vi "SensorInfo.vi"(0 "Serial Number":string, 5 "Family":u16(ring) items=["Iris Slim", "Iris Compact", "Iris xxxx"], 9 "Revision (iteración)":string) -> (4 "Serial Number out":string, 6 "Family out":u16(ring) items=["Iris Slim", "Iris xxxx", "Iris xxxx"], 8 "Part Number out":string, 10 "Revision out":string)   [LabVIEW 2018]
panel:
  in  "Cancel":bool
  in  "OK":bool
  # "Test Information"
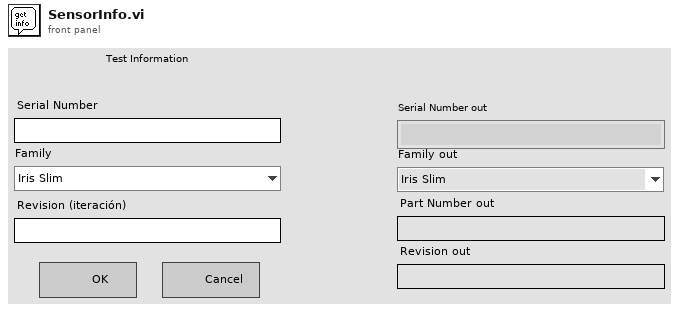
[diagram p1: front panel]
types:
  T1 = enum8{"Enabled", "Disabled", "Disabled and Grayed Out"}
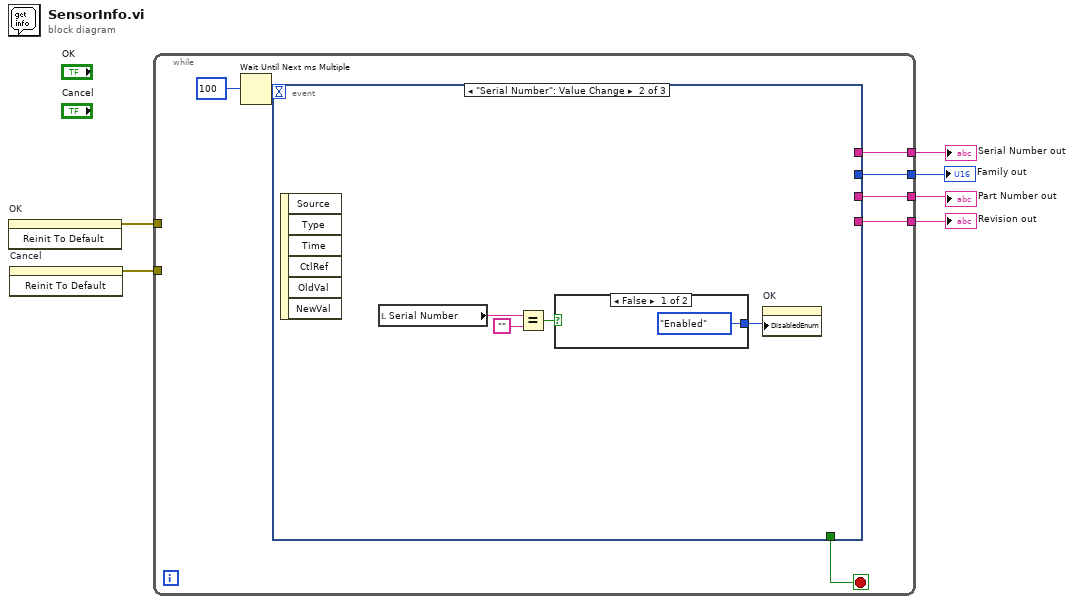
[diagram p0: block diagram]
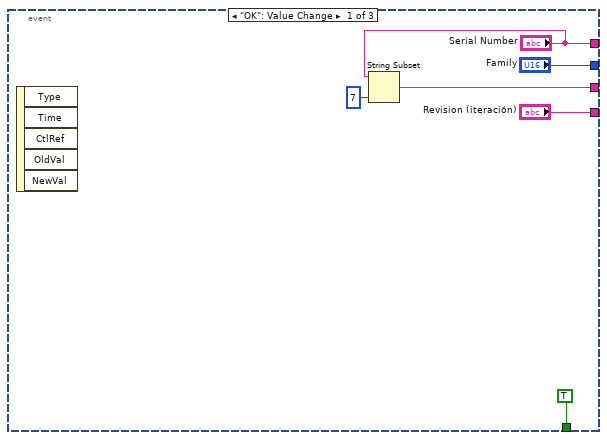
[diagram p2: hidden frame]
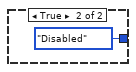
[diagram p3: hidden frame]
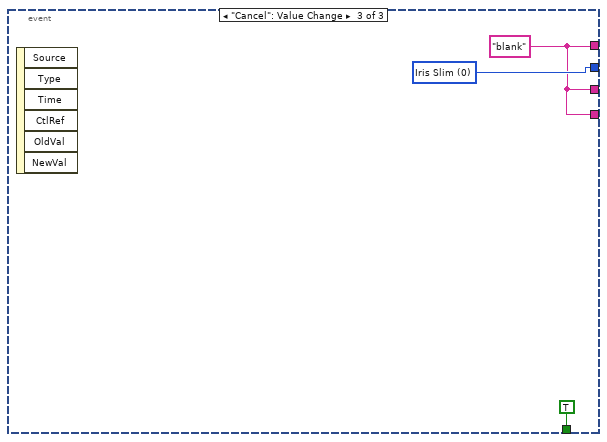
[diagram p4: hidden frame]
diagram:
  n1 = invoke on="OK" class="Bool" method="Reinit To Default"() -> (error out=w5:errorcluster)  [unwired: 3 in, 2 out]
  n2 = invoke on="Cancel" class="Bool" method="Reinit To Default"() -> (error out=w4:errorcluster)  [unwired: 3 in, 2 out]
  n3 = while {
    tunnel: [w12] -> w6
    tunnel: [w11] -> w1
    tunnel: w5 -> [_]
    tunnel: w4 -> [_]
    tunnel: [w8] -> w3
    tunnel: [w7] -> w2
    stop <- w9 stop-if-true
    n4 = Wait Until Next ms Multiple(millisecond multiple=100) -> ()  [unwired: 1 out]
    n5 = event shown="[1] \"Serial Number\": Value Change" {
      selector: _ -> [_ _ _]
      dyn-events: _ -> [_ _ _]
      timeout: _ -> [_ _ _]
      tunnel: [TRUE _ TRUE] -> w9
      tunnel: ["Serial Number" _ w25] -> w12
      tunnel: ["Family" _ w26] -> w11
      tunnel: ["Revision (iteración)" _ w25] -> w8
      tunnel: [w13 _ w25] -> w7
      event "OK": Value Change {
        n6 = event-data() -> ()  [unwired: 6 out]
        n7 = String Subset(string="Serial Number", length (rest)=7 ("length (rest)")) -> (substring=w13:string)  [unwired: 1 in]
      }
      event "Serial Number": Value Change {
        n8 = event-data() -> ()  [unwired: 7 out]
        n9 = local read "Serial Number"() -> (w22:string)
        n10 = Equal?(x=w22, y="") -> (x = y?=w21:bool)
        n11 = case shown="False" w21 {
          tunnel: [T1."Enabled" ("Disabled") T1."Disabled" ("Disabled")] -> w20
          frame False {
          }
          frame True {
          }
        }
        n12 = property on="OK" class="Bool"("DisabledEnum"=w20) -> ()  [unwired: 2 in, 2 out]
      }
      event "Cancel": Value Change {
        w26 = u16 0 items=["Iris Slim", "Iris xxxx", "Iris xxxx"] ("Family out")
        w25 = "blank" ("Name")
        n13 = event-data() -> ()  [unwired: 7 out]
      }
    }
  }
  "Serial Number out" <- w6
  "Revision out" <- w3
  "Part Number out" <- w2
  "Family out" <- w1
